vi "CheckAQHeader.vi"(8 "Error In":errorcluster, 11 "Encoded Data In":u8[](array[numeric])) -> (0 "Error Out":errorcluster, 3 "Header Found":bool)   [LabVIEW 2010]
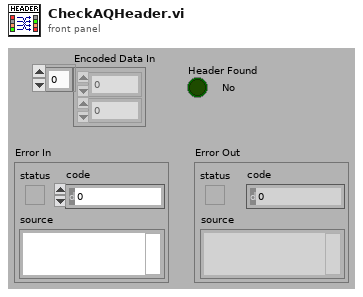
[diagram p1: front panel]
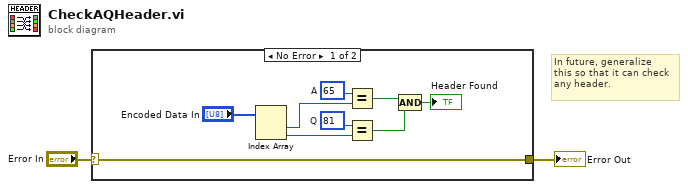
[diagram p0: block diagram]
diagram:
  # "In future, generalize\nthis so that it can check\nany header."
  n1 = case shown="No Error" "Error In" {
    selector: "Error In" -> [w3 w12]
    tunnel: [w3 w12] -> w1
    frame No Error {
      w9 = u8 81  # Q
      w7 = u8 65  # A
      n2 = Index Array(array="Encoded Data In") -> (element #1=w8:u8, element #2=w10:u8)  [unwired: 2 in]
      n3 = Equal?(x=w7, y=w8) -> (x = y?=w6:bool)
      n4 = Equal?(x=w9, y=w10) -> (x = y?=w5:bool)
      n5 = Compound Arithmetic op=AND(w6, w5) -> (→"Header Found":bool)
    }
    frame Error {
    }
  }
  "Error Out" <- w1
